vi "Measuring Example (B).vi"() -> ()   [LabVIEW 2011]
uses:
  C:/Program Files/Metrohm Autolab/Autolab SDK 1.10/EcoChemie.Autolab.Sdk.dll
  EcoChemie.Autolab.Sdk.dll
panel:
  out "PotentialApplied":dbl
  out "Y: WE(1).Current":dbl
  out "X: WE(1).Potential":dbl
  out "XY Graph":cluster{"Y":dbl[], "Y":dbl[]}[](graph)
  in  "Abort":bool
  in  "fileName":string
  out "IsMeasuring":bool
  in  "Save":bool
  in  "start measure":bool
  in  "Stop":bool
  out "IsConnected":bool
  out "error out":errorcluster
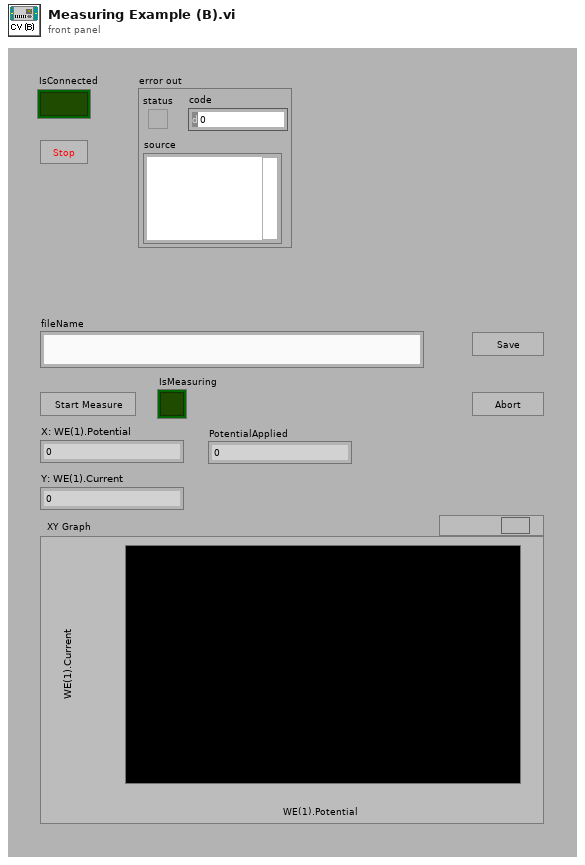
[diagram p1: front panel]
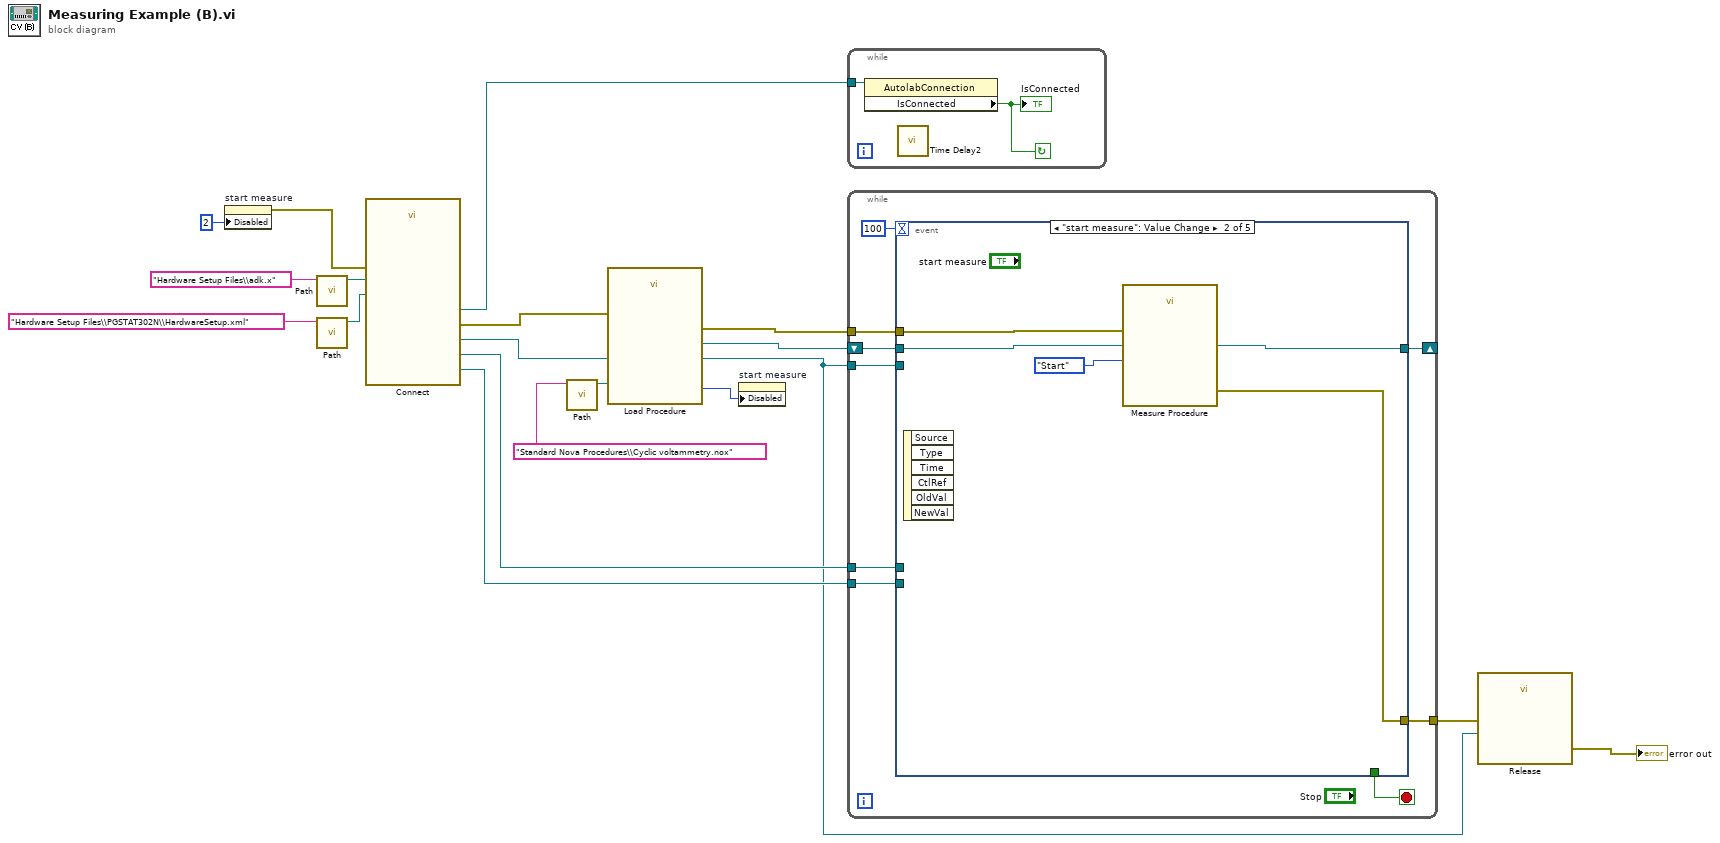
[diagram p0: block diagram]
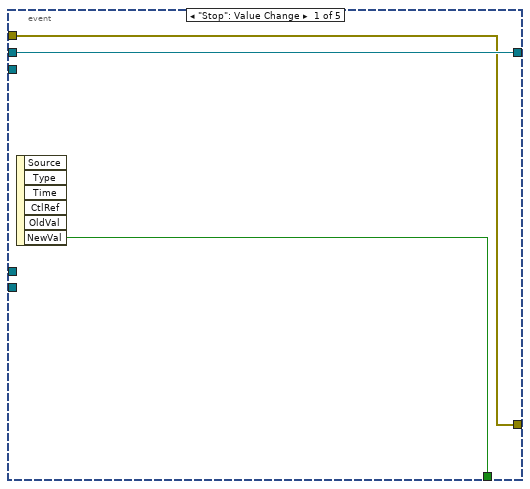
[diagram p2: hidden frame]
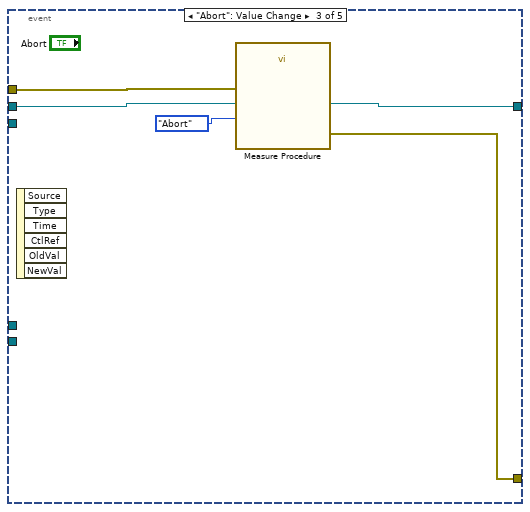
[diagram p3: hidden frame]
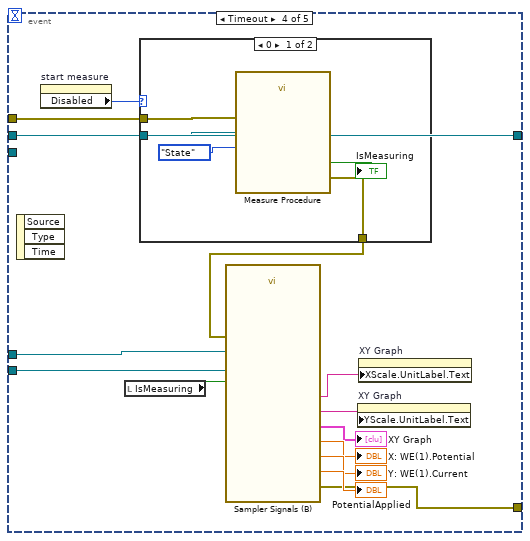
[diagram p4: hidden frame]
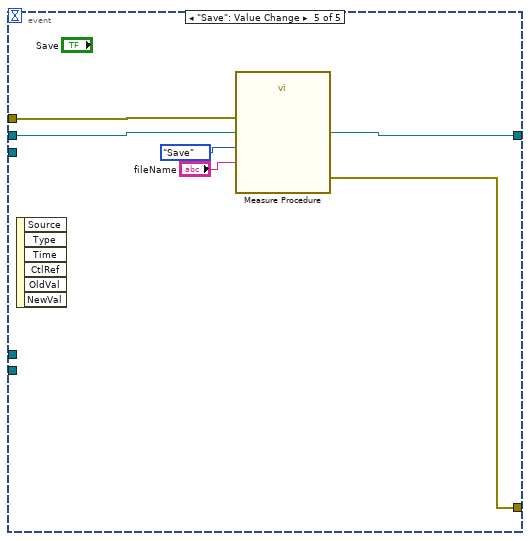
[diagram p6: hidden frame]
diagram:
  n1 = property on="start measure" class="Bool"("Disabled"=u8 2) -> (error out=w1:errorcluster)  [unwired: 2 in, 1 out]
  n2 = call "Path.vi"("name or relative path"="Hardware Setup Files\\adk.x") -> ("appended path"=w14:path)  [unwired: 10 in]
  n3 = call "Path.vi"("name or relative path"="Hardware Setup Files\\PGSTAT302N\\HardwareSetup.xml") -> ("appended path"=w13:path)  [unwired: 10 in]
  n4 = call "Connect.vi"("Embedded Exe File"=w14, "Hardware Setup File"=w13, "error in (no error)"=w1) -> ("Sampler"=w12:refnum<k24>, "AutolabConnection"=w17:refnum<k24>, "instrument"=w7:refnum<k24>, "Ei"=w11:refnum<k24>, "error out"=w8:errorcluster)  [unwired: 5 in, 3 out]
  n5 = call "Path.vi"("name or relative path"="Standard Nova Procedures\\Cyclic voltammetry.nox") -> ("appended path"=w6:path)  [unwired: 10 in]
  n6 = call "Load Procedure.vi"("error in (no error)"=w8, "Procedure"=w6, "Instrument"=w7) -> ("error out"=w4:errorcluster, "Numeric"=w5:i32, "LoadProcedure"=w3:refnum<k24>)  [unwired: 5 in, 1 out]
  n7 = property on="start measure" class="Bool"("Disabled"=w5) -> ()  [unwired: 2 in, 2 out]
  n8 = while {
    tunnel: w17 -> [w19]
    stop <- w20 continue-if-true
    n9 = property class="AutolabConnection"(reference=w19) -> ("IsConnected"=w20:bool)  [unwired: 1 in, 2 out]
    "IsConnected" <- w20
    n10 = call "Time Delay2"() -> ()  [unwired: 11 in, 1 out]
  }
  n11 = while {
    tunnel: [w29] -> w10
    tunnel: w4 -> [w28]
    tunnel: w12 -> [w25]
    tunnel: w11 -> [w24]
    shift-right: [w23] -> _
    shift-left: w3 -> [w21]
    tunnel: w7 -> [w22]
    stop <- w27 stop-if-true
    n12 = event shown="[1] \"start measure\": Value Change" {
      selector: _ -> [_ _ _ _ _]
      dyn-events: _ -> [_ _ _ _ _]
      timeout: 100 -> [_ _ _ _ _]
      tunnel: [w30 w34 w38 w41 w64] -> w29
      tunnel: w21 -> [w31 w33 w37 w53 w61]
      tunnel: w28 -> [w30 w36 w39 w54 w65]
      tunnel: [w32 _ _ _ _] -> w27
      tunnel: w25 -> [_ _ _ w43 _]
      tunnel: w24 -> [_ _ _ w42 _]
      tunnel: [w31 w33 w37 w53 w61] -> w23
      tunnel: w22 -> [_ _ _ _ _]
      event "Stop": Value Change {
        n13 = event-data() -> ("NewVal"=w32:bool)  [unwired: 1 in, 5 out]
      }
      event "start measure": Value Change {
        n14 = event-data() -> ()  [unwired: 1 in, 6 out]
        n15 = call "Measure Procedure.vi"("error in"=w36, "Request for procedure"=enum16{"State", "Save", "Abort", "Start"}."Start", "LoadProcedure"=w33) -> ("error out"=w34:errorcluster)  [unwired: 7 in, 1 out]
      }
      event "Abort": Value Change {
        n16 = event-data() -> ()  [unwired: 1 in, 6 out]
        n17 = call "Measure Procedure.vi"("error in"=w39, "Request for procedure"=enum16{"State", "Save", "Abort", "Start"}."Abort", "LoadProcedure"=w37) -> ("error out"=w38:errorcluster)  [unwired: 7 in, 1 out]
      }
      event Timeout {
        n18 = event-data() -> ()  [unwired: 1 in, 3 out]
        n19 = property on="start measure" class="Bool"() -> ("Disabled"=w52:u8)  [unwired: 2 in, 2 out]
        n20 = local read "IsMeasuring"() -> (w45:bool)
        n21 = case shown="0" w52 {
          tunnel: w54 -> [w58 w60]
          tunnel: [w57 w60] -> w44
          tunnel: w53 -> [w55 _]
          frame 0 {
            n22 = call "Measure Procedure.vi"("error in"=w58, "Request for procedure"=enum16{"State", "Save", "Abort", "Start"}."State", "LoadProcedure"=w55) -> ("error out"=w57:errorcluster, "IsMeasuring"=→"IsMeasuring":bool)  [unwired: 7 in]
          }
          frame 1, Default {
          }
        }
        n23 = call "Sampler Signals (B).vi"("Sampler"=w43, "EI"=w42, "measure"=w45, "error in"=w44) -> ("X"=→"X: WE(1).Potential":dbl, "Y"=→"Y: WE(1).Current":dbl, "Signal X"=w46:string, "XY Graph"=→"XY Graph":cluster{"Y":dbl[], "Y":dbl[]}[], "Signal Y"=w47:string, "PotentialApplied"=→"PotentialApplied":dbl, "error out"=w41:errorcluster)  [unwired: 5 in]
        n24 = property on="XY Graph" class="XYGraph (strict)"("YScale.UnitLabel.Text"=w47) -> ()  [unwired: 2 in, 2 out]
        n25 = property on="XY Graph" class="XYGraph (strict)"("XScale.UnitLabel.Text"=w46) -> ()  [unwired: 2 in, 2 out]
      }
      event "Save": Value Change {
        n26 = event-data() -> ()  [unwired: 1 in, 6 out]
        n27 = call "Measure Procedure.vi"("error in"=w65, "fileName"="fileName", "Request for procedure"=enum16{"State", "Save", "Abort", "Start"}."Save", "LoadProcedure"=w61) -> ("error out"=w64:errorcluster)  [unwired: 6 in, 1 out]
      }
    }
  }
  n28 = call "Release.vi"("error in (no error)"=w10, "Instrument"=w7) -> ("error out"=→"error out":errorcluster)  [unwired: 9 in]
